vi "filter_wheel.vi"() -> ()   [LabVIEW 2015]
uses:
  Instance           1 14Saved   Sample .vi
panel:
  in  "OpenClose":bool
  in  "ShowDialog":bool
  in  "MoveDown":bool
  in  "MoveUp":bool
  out "Position":i16
  in  "SelectBaudRate":bool
  in  "SelectComPort":bool
  out "ComPort":string
  out "BaudRate":i32
  in  "stop":bool
  in  "FW102":refnum<k7>(container)
  # "6 -> open\n1-> closed"
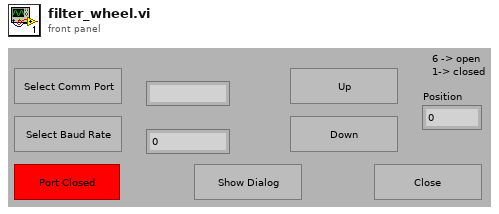
[diagram p1: front panel]
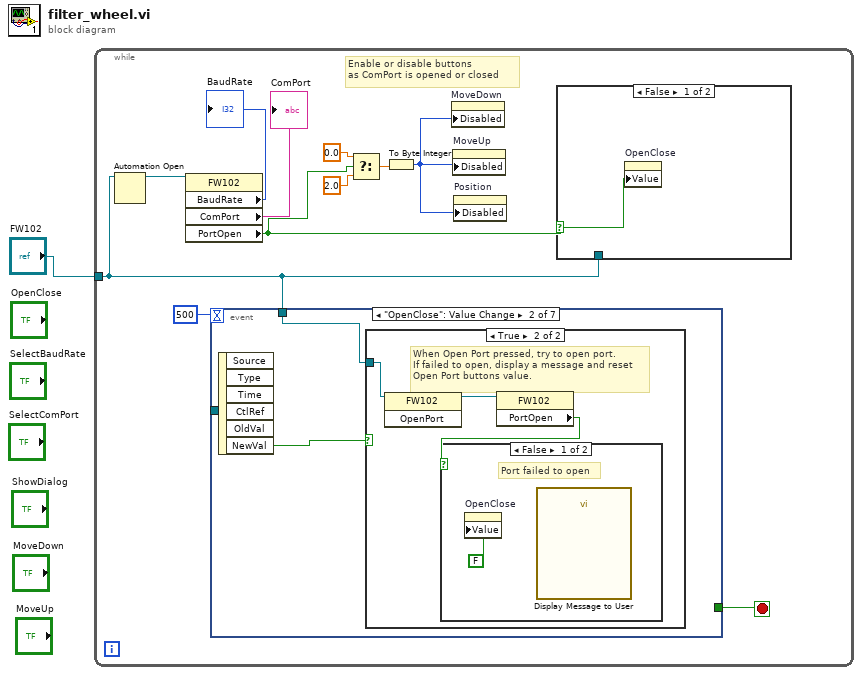
[diagram p0: block diagram]
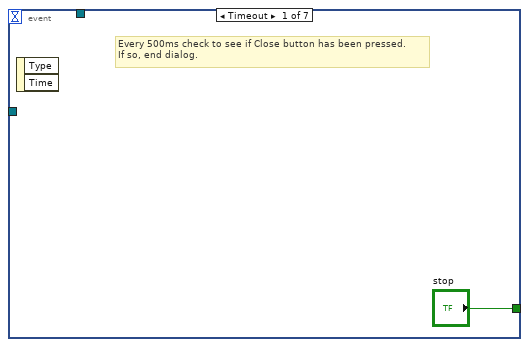
[diagram p2: hidden frame]
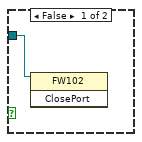
[diagram p3: hidden frame]
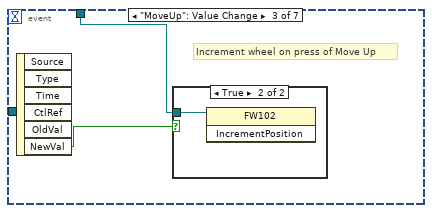
[diagram p5: hidden frame]
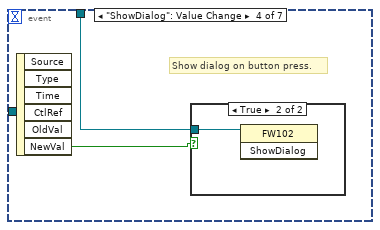
[diagram p7: hidden frame]
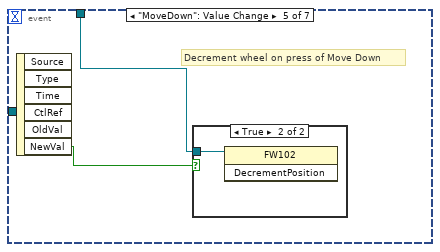
[diagram p9: hidden frame]
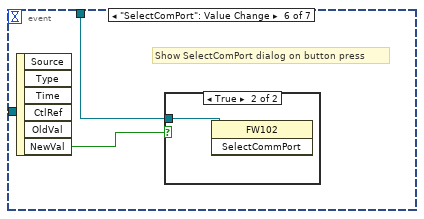
[diagram p11: hidden frame]
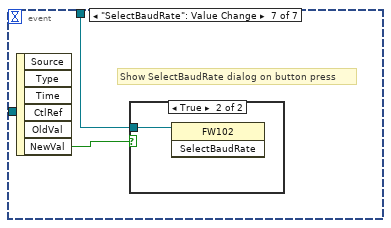
[diagram p13: hidden frame]
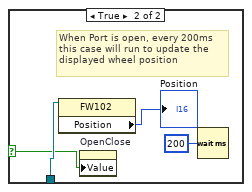
[diagram p15: hidden frame]
diagram:
  n1 = while {
    tunnel: "FW102" -> [w7]
    stop <- w9 stop-if-true
    # "Enable or disable buttons \nas ComPort is opened or closed"
    n2 = Automation Open(Automation Refnum=w7) -> (Automation Refnum=w12:refnum<k7>)  [unwired: 1 in, 3 out]
    n3 = property class="FW102"(reference=w12) -> ("BaudRate"=→"BaudRate":i32, "ComPort"=→"ComPort":string, "PortOpen"=w3:bool)  [unwired: 1 in, 2 out]
    n4 = event shown="[1] \"OpenClose\": Value Change" {
      selector: _ -> [_ _ _ _ _ _ _]
      dyn-events: _ -> [_ _ _ _ _ _ _]
      timeout: 500 -> [_ _ _ _ _ _ _]
      tunnel: [_ w16 _ _ _ _ _] -> _
      tunnel: w7 -> [_ w14 w23 w26 w29 w32 w35]
      tunnel: ["stop" _ _ _ _ _ _] -> w9
      event Timeout {
        # "Every 500ms check to see if Close button has been pressed.\nIf so, end dialog."
        n5 = event-data() -> ()  [unwired: 3 out]
      }
      event "OpenClose": Value Change {
        n6 = event-data() -> ("CtlRef"=w16:refnum<vi>, "NewVal"=w15:bool)  [unwired: 5 out]
        n7 = case shown="True" w15 {
          tunnel: w14 -> [w17 w20]
          frame False {
            n8 = invoke class="FW102" method="ClosePort"(reference=w17) -> ()  [unwired: 2 in, 3 out]
          }
          frame True {
            # "When Open Port pressed, try to open port.\nIf failed to open, display a message and reset\nOpen Port buttons value."
            n9 = invoke class="FW102" method="OpenPort"(reference=w20) -> (reference out=w19:refnum<k7>)  [unwired: 2 in, 2 out]
            n10 = property class="FW102"(reference=w19) -> ("PortOpen"=w18:bool)  [unwired: 1 in, 2 out]
            n11 = case shown="False" w18 {
              frame False {
                # "Port failed to open"
                n12 = property on="OpenClose" class="Bool (strict)"("Value"=FALSE ("OpenClose")) -> ()  [unwired: 2 in, 2 out]
                n13 = call "Display Message to User"() -> ()  [unwired: 3 in, 9 out]
              }
              frame True {
                # "Port opened ok, do nothing."
              }
            }
          }
        }
      }
      event "MoveUp": Value Change {
        # "Increment wheel on press of Move Up"
        n14 = event-data() -> ("NewVal"=w22:bool)  [unwired: 6 out]
        n15 = case shown="True" w22 {
          tunnel: w23 -> [_ w24]
          frame False {
          }
          frame True {
            n16 = invoke class="FW102" method="IncrementPosition"(reference=w24) -> ()  [unwired: 2 in, 3 out]
          }
        }
      }
      event "ShowDialog": Value Change {
        # "Show dialog on button press."
        n17 = event-data() -> ("NewVal"=w25:bool)  [unwired: 6 out]
        n18 = case shown="True" w25 {
          tunnel: w26 -> [_ w27]
          frame False {
          }
          frame True {
            n19 = invoke class="FW102" method="ShowDialog"(reference=w27) -> ()  [unwired: 2 in, 3 out]
          }
        }
      }
      event "MoveDown": Value Change {
        # "Decrement wheel on press of Move Down"
        n20 = event-data() -> ("NewVal"=w28:bool)  [unwired: 6 out]
        n21 = case shown="True" w28 {
          tunnel: w29 -> [_ w30]
          frame False {
          }
          frame True {
            n22 = invoke class="FW102" method="DecrementPosition"(reference=w30) -> ()  [unwired: 2 in, 3 out]
          }
        }
      }
      event "SelectComPort": Value Change {
        # "Show SelectComPort dialog on button press"
        n23 = event-data() -> ("NewVal"=w31:bool)  [unwired: 6 out]
        n24 = case shown="True" w31 {
          tunnel: w32 -> [_ w33]
          frame False {
          }
          frame True {
            n25 = invoke class="FW102" method="SelectCommPort"(reference=w33) -> ()  [unwired: 2 in, 3 out]
          }
        }
      }
      event "SelectBaudRate": Value Change {
        # "Show SelectBaudRate dialog on button press"
        n26 = event-data() -> ("NewVal"=w34:bool)  [unwired: 6 out]
        n27 = case shown="True" w34 {
          tunnel: w35 -> [_ w36]
          frame False {
          }
          frame True {
            n28 = invoke class="FW102" method="SelectBaudRate"(reference=w36) -> ()  [unwired: 2 in, 3 out]
          }
        }
      }
    }
    n29 = Select(t=0.0, s=w3, f=2.0) -> (s? t:f=w4:dbl)
    n30 = To Byte Integer(number=w4) -> (8bit integer=w2:i8)
    n31 = property on="MoveDown" class="Bool (strict)"("Disabled"=w2) -> ()  [unwired: 2 in, 2 out]
    n32 = property on="MoveUp" class="Bool (strict)"("Disabled"=w2) -> ()  [unwired: 2 in, 2 out]
    n33 = property on="Position" class="DigNum (strict)"("Disabled"=w2) -> ()  [unwired: 2 in, 2 out]
    n34 = case shown="False" w3 {
      selector: w3 -> [w37 w38]
      tunnel: w7 -> [_ w41]
      frame False {
        n35 = property on="OpenClose" class="Bool (strict)"("Value"=w37) -> ()  [unwired: 2 in, 2 out]
      }
      frame True {
        # "When Port is open, every 200ms\nthis case will run to update the\ndisplayed wheel position"
        n36 = property class="FW102"(reference=w41) -> ("Position"=→"Position":i16)  [unwired: 1 in, 2 out]
        n37 = property on="OpenClose" class="Bool (strict)"("Value"=w38) -> ()  [unwired: 2 in, 2 out]
        n38 = Wait (ms)(milliseconds to wait=u32 200) -> ()  [unwired: 1 out]
      }
    }
  }
